vi "getActiveChannels_All.vi"(11 "showAll array":refnum<vi>[](array[refnum])) -> (3 "active Channels":i32[](array[numeric]))   [LabVIEW 2011]
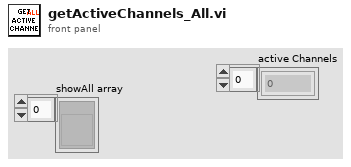
[diagram p1: front panel]
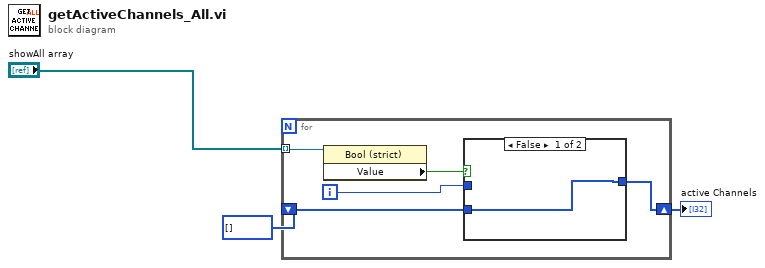
[diagram p0: block diagram]
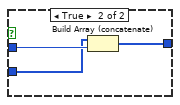
[diagram p2: hidden frame]
diagram:
  n1 = for {
    tunnel: "showAll array" -> [w8] mode=indexing
    shift-right: [w5] -> w1
    shift-left: i32[] [] -> [w4]
    i -> [w6]
    n2 = property class="Bool (strict)"(reference=w8) -> ("Value"=w7:bool)  [unwired: 1 in, 2 out]
    n3 = case shown="False" w7 {
      tunnel: w6 -> [_ w12]
      tunnel: [w9 w11] -> w5
      tunnel: w4 -> [w9 w10]
      frame False {
      }
      frame True {
        n4 = Build Array (concatenate)(w10, w12) -> (w11:i32[])
      }
    }
  }
  "active Channels" <- w1
